vi "PH_gentec_Powermeter.set wanted Settings.vi"(0 "i ref in":refnum<vi>, 2 "VISA resource in":refnum<visa-resource-name>, 5 "error in":errorcluster) -> (13 "Timeout":bool, 14 "i ref out":refnum<vi>, 17 "Error Messages":string, 18 "Device Error out":errorcluster, 19 "error out":errorcluster)   [LabVIEW 2014, in "PH_gentec_Powermeter.lvlib"]
doc: "This VI sets the device to the wanted settings."
uses:
  PH_gentec_Powermeter.lvlib
  non_GPL/instr.lib/gentec-SOLO-PE/gentec-SOLO-PE - Driver.lvlib
  PH_Powermeter_BaseClass/PH_Powermeter_BaseClass.lvlib
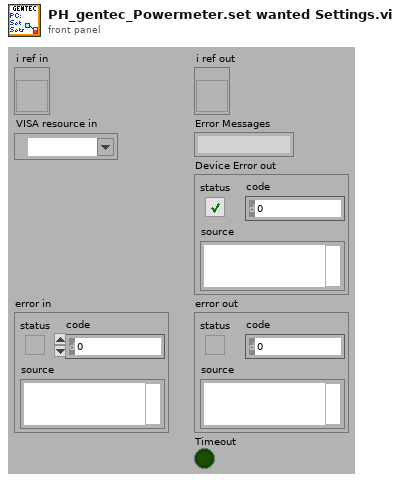
[diagram p1: front panel]
types:
  T1 = typedef "gentec-SOLO-PE - Driver.lvlib/gentec-SOLO-PE.Configuration Values.ctl" = cluster{"Head Type":string, "Head Version":u32, "Serial Number":string, "Calibration Sensitivity":dbl, "Default Wavelength":u32, "Active Sensitivity":dbl, "Active Wavelength":u32, "Scale Min Power":u32, "Scale Max Power":u32, "Scale Min Energy":T2, "Scale Max Energy":T2, "Current Scale":T2, "Calo Mode":bool, "Anticipation":bool, "External Trig":bool, "Trig Level":dbl, "Zero Offset":dbl, "Multiplier 1":dbl, "Offset 1":dbl, "Multiplier 2":dbl, "Offset 2":dbl, "Max Power (Joulemeter)":dbl, "Max energy (Joulemeter)":dbl, "Currently Logging":bool, "Analog Out Active":bool, "Resolution":dbl, "Currently Calculating Stats":bool, "High-Resolution Display":bool, "Scale Min Wavelenght":u32, "Scale Max Wavelenght":u32, "Upper Bound":dbl, "Lower Bond":dbl, "Reference Value":dbl, "Thresholds Active":bool, "Fail":bool}
  T2 = typedef "gentec-SOLO-PE - Driver.lvlib/gentec-SOLO-PE.Scale.ctl" = u32
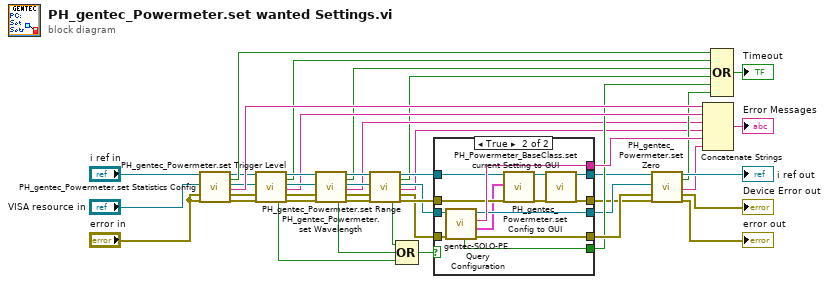
[diagram p0: block diagram]
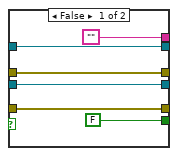
[diagram p2: hidden frame]
diagram:
  n1 = call "PH_gentec_Powermeter.set Statistics Config.vi"("i ref in"="i ref in", "VISA resource in"="VISA resource in", "Device error in"="error in", "error in"="error in") -> ("i ref out"=w18:refnum<vi>, "Timeout"=w32:bool, "VISA resource out"=w17:refnum<visa-resource-name>, "Error Messages"=w34:string, "Device error out"=w16:errorcluster, "error out"=w15:errorcluster)  [unwired: 10 in]
  n2 = call "PH_gentec_Powermeter.set Trigger Level.vi"("i ref in"=w18, "VISA resource in"=w17, "Device error in"=w16, "error in"=w15) -> ("Settings changed"=w28:bool, "i ref out"=w40:refnum<vi>, "Timeout"=w30:bool, "VISA resource out"=w39:refnum<visa-resource-name>, "Error Message"=w29:string, "Device error out"=w36:errorcluster, "error out"=w41:errorcluster)  [unwired: 9 in]
  n3 = call "PH_gentec_Powermeter.set Wavelength.vi"("i ref in"=w40, "VISA resource in"=w39, "Device error in"=w36, "error in"=w41) -> ("Settings changed?"=w27:bool, "i ref out"=w14:refnum<vi>, "Timeout"=w4:bool, "VISA resource out"=w12:refnum<visa-resource-name>, "Error Message"=w5:string, "Device error out"=w11:errorcluster, "error out"=w10:errorcluster)  [unwired: 9 in]
  n4 = call "PH_gentec_Powermeter.set Range.vi"("i ref in"=w14, "VISA resource in"=w12, "Device error in"=w11, "error in"=w10) -> ("Settings changed?"=w6:bool, "i ref out"=w13:refnum<vi>, "Timeout"=w3:bool, "VISA resource out"=w7:refnum<visa-resource-name>, "Error Message"=w2:string, "Device error out"=w8:errorcluster, "error out"=w9:errorcluster)  [unwired: 9 in]
  n5 = Compound Arithmetic op=OR(w6, w27, w28) -> (w1:bool)
  n6 = case shown="True" w1 {
    tunnel: w8 -> [w47 w63]
    tunnel: [w47 w62] -> w26
    tunnel: ["" w61] -> w25
    tunnel: [FALSE ("Timeout") w60] -> w24
    tunnel: w7 -> [w48 w59]
    tunnel: [w48 w58] -> w23
    tunnel: w9 -> [w49 w57]
    tunnel: [w49 w53] -> w22
    tunnel: w13 -> [w50 w55]
    tunnel: [w50 w51] -> w21
    frame False {
    }
    frame True {
      n7 = call "gentec-SOLO-PE.Query Configuration.vi"("error in (no error)"=w63, "VISA Refnum in"=w59) -> ("error out"=w62:errorcluster, "Configuration"=w54:T1, "Error"=w61:string, "VISA Refnum out"=w58:refnum<visa-resource-name>, "Timeout"=w60:bool)  [unwired: 5 in]
      n8 = call "PH_gentec_Powermeter.set Config to GUI.vi"("i ref in"=w55, "Configuration Values"=w54, "error in"=w57) -> ("i ref out"=w52:refnum<vi>, "error out"=w56:errorcluster)  [unwired: 15 in]
      n9 = call "PH_Powermeter_BaseClass.set current Setting to GUI.vi"("VI in"=w52, "error in (no error)"=w56) -> ("VI out"=w51:refnum<vi>, "error out"=w53:errorcluster)  [unwired: 16 in]
    }
  }
  n10 = call "PH_gentec_Powermeter.set Zero.vi"("i ref in"=w21, "VISA resource in"=w23, "Device error in"=w26, "error in"=w22) -> ("i ref out"=→"i ref out":refnum<vi>, "Timeout"=w19:bool, "Error Message"=w20:string, "Device error out"=→"Device Error out":errorcluster, "error out"=→"error out":errorcluster)  [unwired: 10 in, 1 out]
  n11 = Concatenate Strings(w34, w29, w5, w2, w25, w20) -> (→"Error Messages":string)
  n12 = Compound Arithmetic op=OR(w32, w30, w4, w3, w24, w19) -> (→"Timeout":bool)
